vi "Configure 16 Point Linearization Point Values.vi"(6 "Points (1)":u8=1 min=1 max=14, 7 "Unit Address (1)":u8=1, 8 "error in (no error)":errorcluster, 9 "Output Value of Point (0)":i32, 10 "Input Value of Point (0)":i32, 11 "VISA resource name":refnum<visa-resource-name>) -> (0 "error out":errorcluster, 3 "VISA resource name out":refnum<visa-resource-name>)   [LabVIEW 2014, in "Eurotherm 35xx Series.lvlib"]
doc: "This VI configure values of selected point of 16 Point Linearisation."
uses:
  <instrlib>/Eurotherm 35xx Series/Eurotherm 35xx Series.lvlib
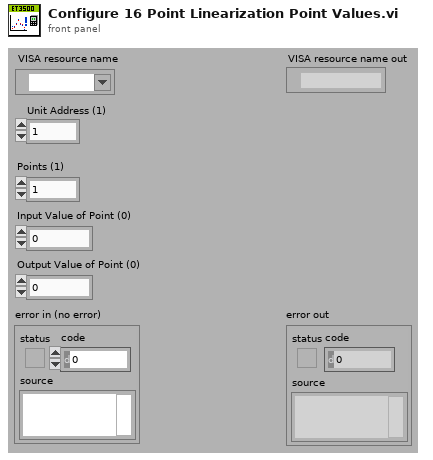
[diagram p1: front panel]
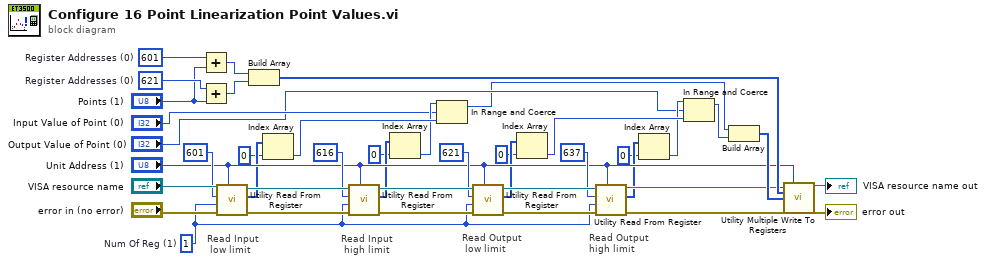
[diagram p0: block diagram]
diagram:
  w22 = u16 1  # Num Of Reg (1)
  w37 = 601  # Register Addresses (0)
  w39 = 621  # Register Addresses (0)
  # "Read Output\nhigh limit"
  # "Read Output\n low limit"
  # "Read Input\n high limit"
  # "Read Input\n low limit"
  n1 = Add(x=w37, y="Points (1)") -> (x+y=w36:i32)
  n2 = Add(x=w39, y="Points (1)") -> (x+y=w35:i32)
  n3 = call <instrlib>:"Utility Read From Register.vi"("Unit Address (1)"="Unit Address (1)", "error in (no error)"="error in (no error)", "Num Of Reg (1)"=w22, "Register Address (0)"=u16 601, "VISA resource name"="VISA resource name") -> ("error out"=w27:errorcluster, "Data"=w16:i16[], "VISA resource name out"=w31:refnum<visa-resource-name>)  [unwired: 4 in]
  n4 = Build Array(w36, w35) -> (w34:i32[])
  n5 = Index Array(array=w16, index=0) -> (element=w8:i16)
  n6 = call <instrlib>:"Utility Read From Register.vi"("Unit Address (1)"="Unit Address (1)", "error in (no error)"=w27, "Num Of Reg (1)"=w22, "Register Address (0)"=u16 616, "VISA resource name"=w31) -> ("error out"=w26:errorcluster, "Data"=w15:i16[], "VISA resource name out"=w30:refnum<visa-resource-name>)  [unwired: 4 in]
  n7 = Index Array(array=w15, index=0) -> (element=w7:i16)
  n8 = In Range and Coerce(upper limit=w7, x="Input Value of Point (0)", lower limit=w8) -> (coerced(x)=w2:i32)  [unwired: 1 out]
  n9 = call <instrlib>:"Utility Read From Register.vi"("Unit Address (1)"="Unit Address (1)", "error in (no error)"=w26, "Num Of Reg (1)"=w22, "Register Address (0)"=u16 621, "VISA resource name"=w30) -> ("error out"=w25:errorcluster, "Data"=w14:i16[], "VISA resource name out"=w29:refnum<visa-resource-name>)  [unwired: 4 in]
  n10 = Index Array(array=w14, index=0) -> (element=w6:i16)
  n11 = call <instrlib>:"Utility Read From Register.vi"("Unit Address (1)"="Unit Address (1)", "error in (no error)"=w25, "Num Of Reg (1)"=w22, "Register Address (0)"=u16 637, "VISA resource name"=w29) -> ("error out"=w24:errorcluster, "Data"=w13:i16[], "VISA resource name out"=w23:refnum<visa-resource-name>)  [unwired: 4 in]
  n12 = Index Array(array=w13, index=0) -> (element=w5:i16)
  n13 = In Range and Coerce(upper limit=w5, x="Output Value of Point (0)", lower limit=w6) -> (coerced(x)=w1:i32)  [unwired: 1 out]
  n14 = Build Array(w2, w1) -> (w33:i32[])
  n15 = call <instrlib>:"Utility Multiple Write To Registers.vi"("VISA resource name"=w23, "Unit Address (1)"="Unit Address (1)", "Registers Addresses (0)"=w34, "Data (0)"=w33, "error in (no error)"=w24) -> ("VISA resource name out"=→"VISA resource name out":refnum<visa-resource-name>, "error out"=→"error out":errorcluster)  [unwired: 9 in]
